vi "oax_Config TIO and DSA Channels (MCM).vi"(0 "DAQ Config":T7 {"probe angle [deg]" max=360; "pregain" format="%.2f"; "IEPE" items=["On", "Off", "None"]; "coupling" items=["DC", "AC"]; "engineering units" items=["custom..."=0, "V"=1, "A"=21, "C"=30, "pC"=31, "s"=32, "-"=29, "Pa"=2, "N"=20, "g"=3, "m/s^2"=4, "m/s"=5, "m"=6, "mm/s"=12, "mm"=13, "micron/s"=14, "micron"=15, "in/s^2"=7, "in/s"=8, "in"=9, "mil/s"=10, "mil"=11, "rad/s^2"=16, "rad/s"=17, "rad"=18, "deg/s^2"=26, "deg/s"=27, "deg"=28, "RPM"=22, "cycle/s^2"=23, "Hz"=24, "cycle"=25, "strain"=19]; "sensor sensitivity (mV/EU)" format="%.2f"; "dB reference" format="%.1e"}, 1 "rotating direction":u16(ring) items=["CCW", "CW"], 2 "Tacho Pulse Edge":i32, 3 "Slave Slot Number":i32(ring) caption="PXI Slot Number" items=["Slot 3", "Slot 4", "Slot 5", "Slot 6", "Slot 7", "Slot 8", "Slot 9", "Slot 10", "Slot 11", "Slot 12", "Slot 13", "Slot 14", "Slot 15", "Slot 16"], 4 "DSA device type":T6 items=["4472"=0, "4474"=10, "4461"=1, "4462"=11, "4464"=12, "449x"=6, "9232"=7, "9233"=2, "9234"=3, "9229"=4, "9239"=5], 5 "error in (no error)":errorcluster, 6 "sample rate":dbl=1000.0 format="%0.2f", 7 "Counter(s)":tag="cDAQ4/_ctr0", 8 "max value":dbl=5.0 format="%0.2f", 9 "PFI line (Gate)":tag, 10 "min value":dbl=-5.0 format="%0.2f") -> (11 "channel name":string[](array[string]), 13 "channel info":T3[](array[typedef]) {"pregain" format="%.2f"; "weighting filter" items=["Linear", "A-weighting", "B-weighting", "C-weighting", "ITU-R 468-4", "Dolby", "CCITT", "C-message", "Wb", "Wc", "Wd", "We", "Wf", "Wh", "Wj", "Wk", "Wm", "AES17 20 kHz lowpass", "AES17 40 kHz lowpass", "AES17 20 kHz highpass", "AES17 40 kHz highpass"]; "dB reference" format="%^.1e"; "engineering units" items=["custom..."=0, "V"=1, "A"=21, "C"=30, "pC"=31, "s"=32, "-"=29, "Pa"=2, "N"=20, "g"=3, "m/s^2"=4, "m/s"=5, "m"=6, "mm/s"=12, "mm"=13, "micron/s"=14, "micron"=15, "in/s^2"=7, "in/s"=8, "in"=9, "mil/s"=10, "mil"=11, "rad/s^2"=16, "rad/s"=17, "rad"=18, "deg/s^2"=26, "deg/s"=27, "deg"=28, "RPM"=22, "cycle/s^2"=23, "Hz"=24, "cycle"=25, "strain"=19]; "sensor sensitivity" format="%#_5f"}, 14 "DSA task out":refnum<k21>, 15 "TIO task out":refnum<k21>, 16 "channel properties":T1[](array[typedef]) {"probe angle [deg]" max=360; "direction" items=["CCW", "CW"]}, 17 "synchronization type":u16(ring) items=["by sharing sample clock", "by using reference clock"], 18 "device info":T2, 19 "error out":errorcluster)   [LabVIEW 2017]
doc: "Configures DAQ channel properties based on the user input and starts the DAQmx task."
uses:
  <vilib>/addons/Sound and Vibration/Order Analysis/Example Support/sub VIs/OAXML_DSA MCM DAQ Config.ctl
  <vilib>/addons/_NISVFA/_Shared subVIs/Controls/svc_Engineering Units Text Ring.ctl
  <vilib>/addons/Sound and Vibration/Order Analysis/Example Support/sub VIs/OAXML_DSA Device Type.ctl
  <vilib>/addons/_NISVFA/_Shared subVIs/Controls/svc_Channel Info.ctl
  <vilib>/addons/_NISVFA/_Shared subVIs/Controls/svc_Weighting Filter Text Ring.ctl
  <vilib>/addons/Sound and Vibration/Order Analysis/Data Presentation/SubVIs/OAT MCM Channel Property.ctl
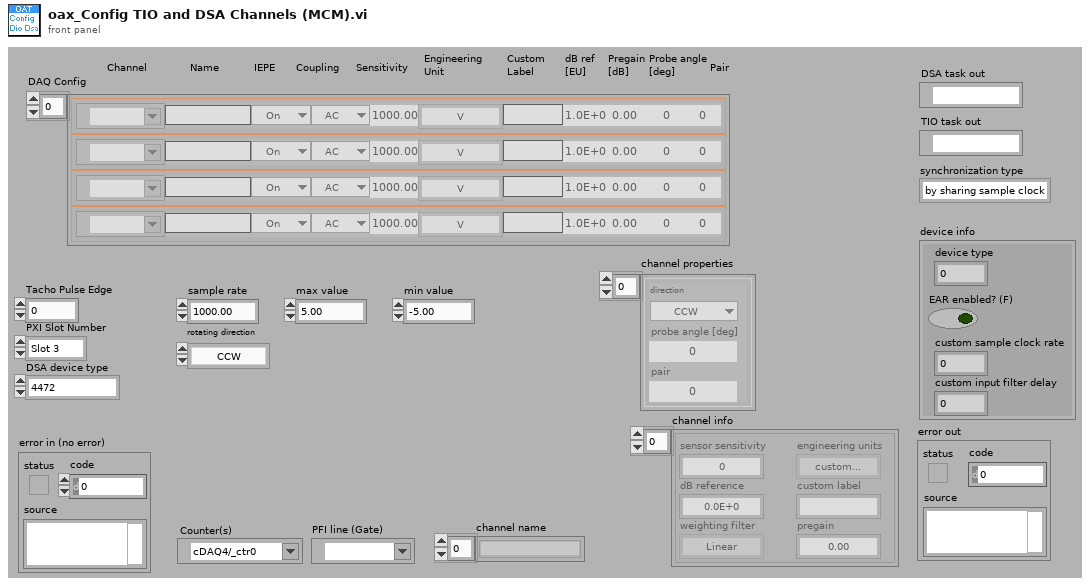
[diagram p1: front panel]
types:
  T1 = typedef "OAT MCM Channel Property.ctl" = cluster{"direction":u16, "probe angle [deg]":u16, "pair":u16}
  T2 = cluster{"device type":u16, "EAR enabled? (F)":bool, "custom sample clock rate":dbl, "custom input filter delay":dbl}
  T3 = typedef "svc_Channel Info.ctl" = cluster{"sensor sensitivity":dbl, "engineering units":T4, "dB reference":dbl, "custom label":string, "weighting filter":T5, "pregain":dbl}
  T4 = typedef "svc_Engineering Units Text Ring.ctl" = u16
  T5 = typedef "svc_Weighting Filter Text Ring.ctl" = u16
  T6 = typedef "OAXML_DSA Device Type.ctl" = u16
  T7 = typedef "OAXML_DSA MCM DAQ Config.ctl" = cluster{"name":string, "channel":tag, "coupling":u16, "dB reference":sgl, "sensor sensitivity (mV/EU)":dbl, "engineering units":T4, "IEPE":u16, "custom label":string, "pregain":sgl, "probe angle [deg]":u16, "pair":u16}[]
  T8 = typedef "OAXML_DSA DAQ Config.ctl" = cluster{"name":string, "channel":tag, "coupling":u16, "dB reference":sgl, "sensor sensitivity (mV/EU)":dbl, "engineering units":T4, "IEPE":u16, "custom label":string, "pregain":sgl}[]
  T9 = cluster{"DSA device type":u16, "EAR enabled? (F)":bool, "custom sample clock rate":dbl, "custom input filter delay":dbl}
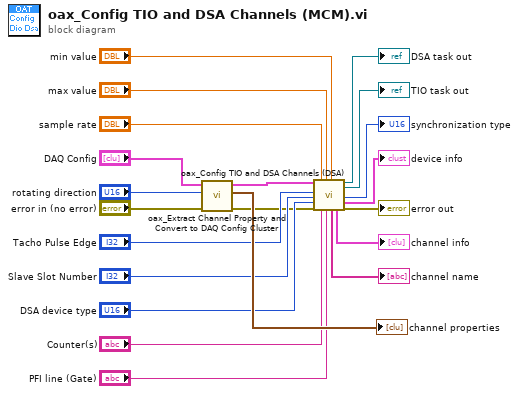
[diagram p0: block diagram]
diagram:
  n1 = call <vilib>:"oax_Extract Channel Property and Convert to DAQ Config Cluster.vi"("error in (no error)"="error in (no error)", "rotating direction"="rotating direction", "MCM DAQ Config"="DAQ Config") -> ("error out"=w10:errorcluster, "channel properties"=→"channel properties":T1[], "DAQ Config"=w14:T8)  [unwired: 6 in]
  n2 = call <vilib>:"oax_Config TIO and DSA Channels (DSA).vi"("DAQ Config"=w14, "Tacho Pulse Edge"="Tacho Pulse Edge", "Slave Slot Number"="Slave Slot Number", "DSA device type"="DSA device type", "error in (no error)"=w10, "sample rate"="sample rate", "Counter(s)"="Counter(s)", "max value"="max value", "PFI line (Gate)"="PFI line (Gate)", "min value"="min value") -> ("channel name"=→"channel name":string[], "channel info"=→"channel info":T3[], "DSA task out"=→"DSA task out":refnum<k21>, "TIO task out"=→"TIO task out":refnum<k21>, "synchronization type"=→"synchronization type":u16, "device info"=→"device info":T9, "error out"=→"error out":errorcluster)  [unwired: 3 in]
